vi "Discretization_DiscretizeAQ.vi"(6 "dT_Seconds":dbl, 9 "ContQ":T1, 10 "ContA":T1, 11 "States":i32) -> (0 "Error":bool, 1 "DiscQ":T1, 3 "DiscA":T1)   [LabVIEW 2019, in "Trajectory_Library.lvlib"]
doc: "Discretizes the given continuous A and Q matrices.\n \nInputs:\n - States -- the number of states.\n - contA -- Continuous system matrix.\n - contQ -- Continuous process noise covariance matrix.\n - dtSeconds -- Discretization timestep.\n\nOutputs:\n - DiscA -- the discrete system matrix\n - DiscQ -- process noise covariance matrix.\n - error -- If TRUE, an error occured."
uses:
  Trajectory_Library.lvlib
  <vilib>/Analysis/Matrix/NI_Matrix.lvlib
  <vilib>/Analysis/Matrix/Numeric/Add/Add - RM,RM.vi
  <vilib>/Analysis/Matrix/Numeric/Multiply/Multiply - RM,R.vi
  <vilib>/Analysis/NI_AALBase.lvlib
  <vilib>/Analysis/baseanly.llb/Real A x B.vi
  <vilib>/Analysis/Matrix/Datatypes/RealMatrix.ctl
panel:
  # "<States,States>"
  # "<States,States>"
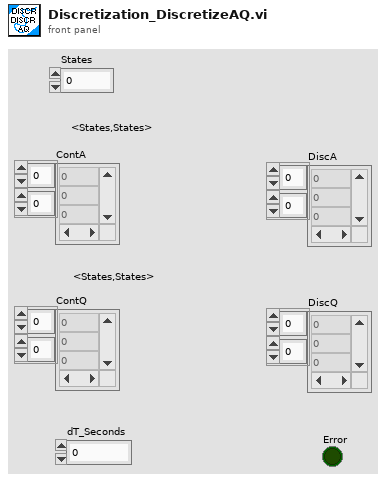
[diagram p1: front panel]
types:
  T1 = typedef "NI_Matrix.lvlib/RealMatrix.ctl" = dbl[][]
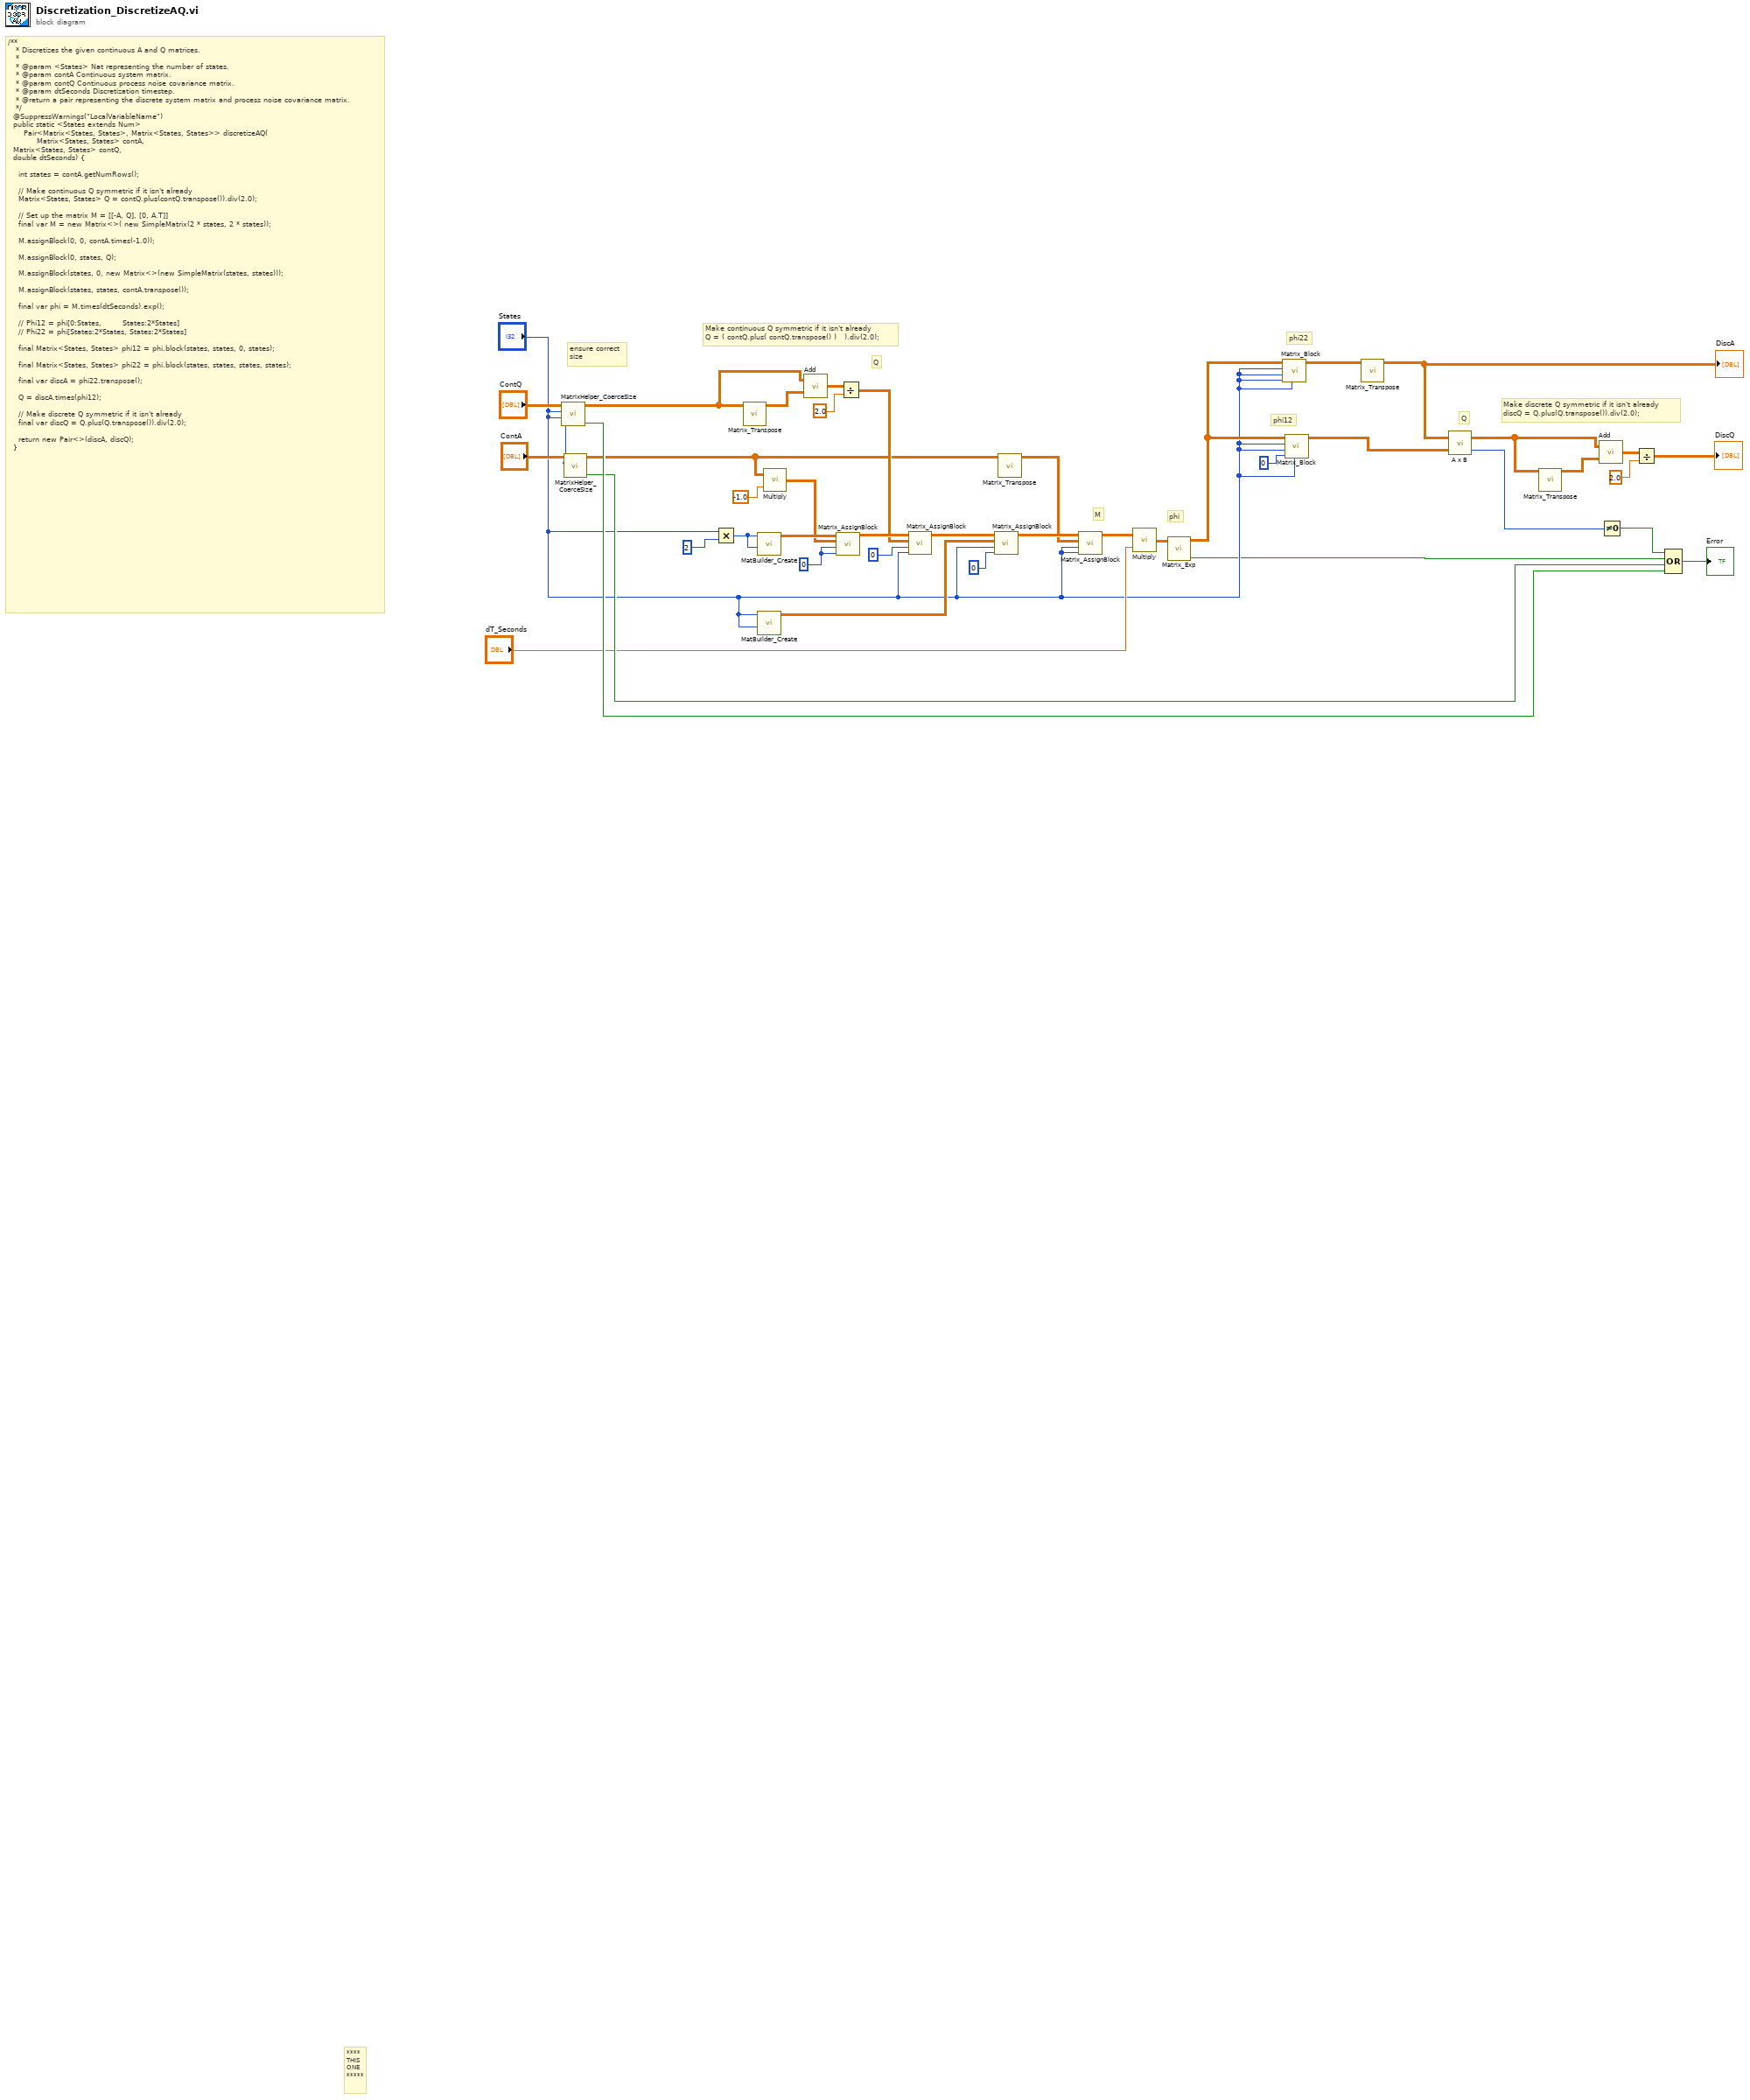
[diagram p0: block diagram]
diagram:
  w26 = 0 ("StartRow")
  # "Make discrete Q symmetric if it isn't already\ndiscQ = Q.plus(Q.transpose()).div(2.0);"
  # "Q"
  # "phi22"
  # "phi12"
  # "phi"
  # "M"
  # "/**\n   * Discretizes the given continuous A and Q matrices.\n   *\n   * @param <States> Nat representing the number of states.\n   * @param contA Continuous system matrix.\n   * @param contQ Continuous process noise covariance matrix.\n   * @param dtSeconds Discretization timestep.\n   * @return a pair representing the discrete system matrix and process noise covariance matrix.\n   */\n  @SuppressWarnings(\"LocalVariableName\")\n  public static <States extends Num>\n      Pair<Matrix<States, States>, Matrix<States, States>> discretizeAQ(\n          \tMatrix<States, States> contA, \n\t\tMatrix<States, States> contQ, \n\t\tdouble dtSeconds) {\n\n    int states = contA.getNumRows();\n\n    // Make continuous Q symmetric if it isn't already\n    Matrix<States, States> Q = contQ.plus(contQ.transpose()).div(2.0);\n\n    // Set up the matrix M = [[-A, Q], [0, A.T]]\n    final var M = new Matrix<>( new SimpleMatrix(2 * states, 2 * states));\n\n    M.assignBlock(0, 0, contA.times(-1.0));\n\n    M.assignBlock(0, states, Q);\n\n    M.assignBlock(states, 0, new Matrix<>(new SimpleMatrix(states, states)));\n\n    M.assignBlock(states, states, contA.transpose());\n\n    final var phi = M.times(dtSeconds).exp();\n\n    // Phi12 = phi[0:States,        States:2*States]\n    // Phi22 = phi[States:2*States, States:2*States]\n\n    final Matrix<States, States> phi12 = phi.block(states, states, 0, states);\n\n    final Matrix<States, States> phi22 = phi.block(states, states, states, states);\n\n    final var discA = phi22.transpose();\n\n    Q = discA.times(phi12);\n\n    // Make discrete Q symmetric if it isn't already\n    final var discQ = Q.plus(Q.transpose()).div(2.0);\n\n    return new Pair<>(discA, discQ);\n  }"
  # "Q"
  # "Make continuous Q symmetric if it isn't already\nQ = ( contQ.plus( contQ.transpose() )   ).div(2.0);"
  # "ensure correct\nsize"
  # "****\nTHIS\nONE\n*****"
  n1 = call "MatrixHelper_CoerceSize.vi"("Columns"="States", "Rows"="States", "input matrix"="ContQ") -> ("Coerced"=w35:bool, "output matrix"=w33:T1)  [unwired: 7 in]
  n2 = call "MatrixHelper_CoerceSize.vi"("Columns"="States", "Rows"="States", "input matrix"="ContA") -> ("Coerced"=w34:bool, "output matrix"=w18:T1)  [unwired: 7 in]
  n3 = Multiply(x="States", y=2) -> (x*y=w30:i32)
  n4 = call "Matrix_Transpose.vi"("input matrix"=w33) -> ("output matrix"=w32:T1)  [unwired: 10 in]
  n5 = call "MatBuilder_Create.vi"("Columns"=w30, "Rows"=w30) -> ("output matrix"=w28:T1)  [unwired: 9 in]
  n6 = call "MatBuilder_Create.vi"("Columns"="States", "Rows"="States") -> ("output matrix"=w21:T1)  [unwired: 9 in]
  n7 = call-poly <vilib>:"Multiply.vi"("Real Scalar c"=-1.0 ("y"), "Real Matrix A"=w18) -> ("A * c"=w27:T1)
  n8 = call-poly <vilib>:"Add.vi"("Real Matrix B"=w32, "Real Matrix A"=w33) -> ("A + B"=w41:T1)
  n9 = call "Matrix_AssignBlock.vi"("StartColumn"=w26, "StartRow"=w26, "Other Matrix"=w27, "input matrix"=w28) -> ("output matrix"=w25:T1)  [unwired: 7 in]
  n10 = Divide(x=w41, y=2.0) -> (x/y=w24:T1)
  n11 = call "Matrix_AssignBlock.vi"("StartColumn"="States", "StartRow"=0, "Other Matrix"=w24, "input matrix"=w25) -> ("output matrix"=w22:T1)  [unwired: 7 in]
  n12 = call "Matrix_AssignBlock.vi"("StartColumn"=0, "StartRow"="States", "Other Matrix"=w21, "input matrix"=w22) -> ("output matrix"=w19:T1)  [unwired: 7 in]
  n13 = call "Matrix_Transpose.vi"("input matrix"=w18) -> ("output matrix"=w17:T1)  [unwired: 10 in]
  n14 = call "Matrix_AssignBlock.vi"("StartColumn"="States", "StartRow"="States", "Other Matrix"=w17, "input matrix"=w19) -> ("output matrix"=w16:T1)  [unwired: 7 in]
  n15 = call-poly <vilib>:"Multiply.vi"("Real Scalar c"="dT_Seconds", "Real Matrix A"=w16) -> ("A * c"=w15:T1)
  n16 = call "Matrix_Exp.vi"("input matrix"=w15) -> ("Error"=w1:bool, "output matrix"=w13:T1)  [unwired: 9 in]
  n17 = call "Matrix_Block.vi"("StartColumn"="States", "StartRow"="States", "Columns"="States", "Rows"="States", "input matrix"=w13) -> ("output matrix"=w10:T1)  [unwired: 6 in]
  n18 = call "Matrix_Block.vi"("StartColumn"="States", "StartRow"=0, "Columns"="States", "Rows"="States", "input matrix"=w13) -> ("output matrix"=w8:T1)  [unwired: 6 in]
  n19 = call "Matrix_Transpose.vi"("input matrix"=w10) -> ("output matrix"=w9:T1)  [unwired: 10 in]
  "DiscA" <- w9
  n20 = call-poly <vilib>:"A x B.vi"("B"=w8, "A"=w9) -> ("error"=w2:i32, "A x B"=w4:T1)
  n21 = call "Matrix_Transpose.vi"("input matrix"=w4) -> ("output matrix"=w5:T1)  [unwired: 10 in]
  n22 = call-poly <vilib>:"Add.vi"("Real Matrix B"=w5, "Real Matrix A"=w4) -> ("A + B"=w7:T1)
  n23 = Not Equal To 0?(x=w2) -> (x != 0?=w39:bool)
  n24 = Divide(x=w7, y=2.0) -> (x/y=→"DiscQ":T1)
  n25 = Compound Arithmetic op=OR(w39, w1, w34, w35) -> (→"Error":bool)
